vi "Return Hex Conversion 05.VI"(9 "Input Array":string[](array[string])) -> (0 "Value str":string, 1 "Calculated Chksum":u8 format="%02x", 2 "Vakue num":dbl format="%.2f", 3 "Description":string, 4 "Checksum Error":bool)   [LabVIEW 2023]
doc: "Converts Neslab return Hex String into comprehensible numbers and functions for display on the main interface."
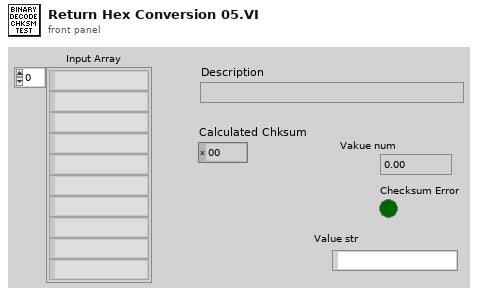
[diagram p1: front panel]
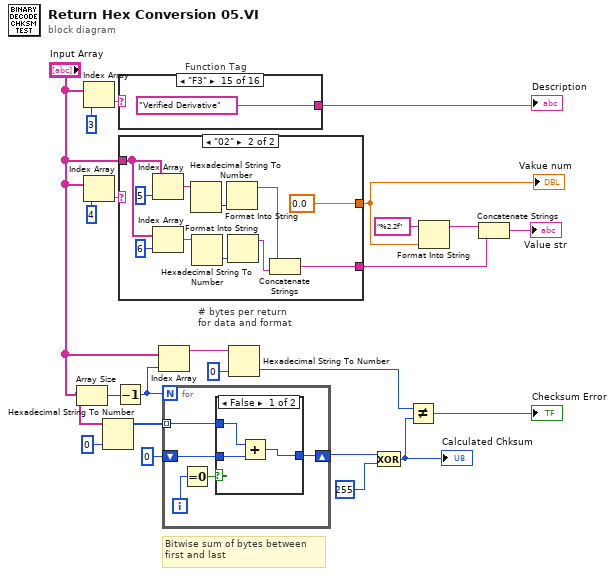
[diagram p0: block diagram]
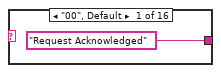
[diagram p3: hidden frame]
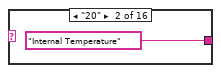
[diagram p4: hidden frame]
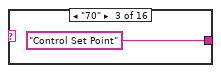
[diagram p5: hidden frame]
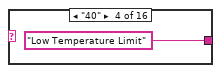
[diagram p6: hidden frame]
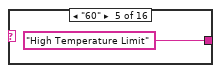
[diagram p7: hidden frame]
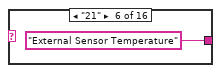
[diagram p8: hidden frame]
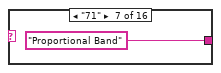
[diagram p9: hidden frame]
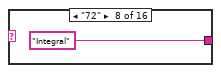
[diagram p10: hidden frame]
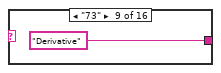
[diagram p11: hidden frame]
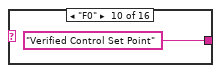
[diagram p12: hidden frame]
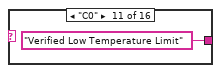
[diagram p13: hidden frame]
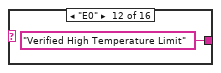
[diagram p14: hidden frame]
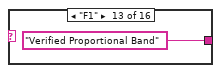
[diagram p15: hidden frame]
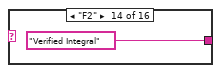
[diagram p16: hidden frame]
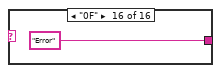
[diagram p17: hidden frame]
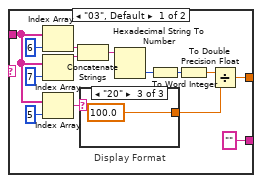
[diagram p18: hidden frame]
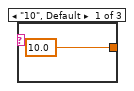
[diagram p19: hidden frame]
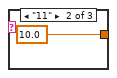
[diagram p20: hidden frame]
diagram:
  # "Bitwise sum of bytes between \nfirst and last"
  # "# bytes per return\nfor data and format"
  # "Function Tag"
  n1 = Array Size(array="Input Array") -> (size(s)=w13:i32)
  n2 = Index Array(array="Input Array", index=3 ("Index")) -> (element=w21:string)
  n3 = Index Array(array="Input Array", index=4 ("Index")) -> (element=w20:string)
  n4 = Hexadecimal String To Number(string="Input Array", default (0uL)=u8 0 ("default (0 U32)")) -> (number=w12:u8[])  [unwired: 1 in, 1 out]
  n5 = Decrement(x=w13) -> (x-1=w7:i32)
  n6 = case shown="\"F3\"" w21 {
    tunnel: ["Request Acknowledged" "Internal Temperature" "Control Set Point" "Low Temperature Limit" "High Temperature Limit" "External Sensor Temperature" "Proportional Band" "Integral" "Derivative" "Verified Control Set Point" "Verified Low Temperature Limit" "Verified High Temperature Limit" "Verified Proportional Band" "Verified Integral" "Verified Derivative" "Error"] -> w17
    frame "00", Default {
    }
    frame "20" {
    }
    frame "70" {
    }
    frame "40" {
    }
    frame "60" {
    }
    frame "21" {
    }
    frame "71" {
    }
    frame "72" {
    }
    frame "73" {
    }
    frame "F0" {
    }
    frame "C0" {
    }
    frame "E0" {
    }
    frame "F1" {
    }
    frame "F2" {
    }
    frame "F3" {
    }
    frame "0F" {
    }
  }
  "Description" <- w17
  n7 = case shown="\"02\"" w20 {
    tunnel: [w46 0.0] -> w15
    tunnel: ["" w65] -> w16
    tunnel: "Input Array" -> [w45 w57]
    frame "03", Default {
      # "Display Format"
      n8 = Index Array(array=w45, index=6 ("Index")) -> (element=w43:string)
      n9 = Index Array(array=w45, index=7 ("Index")) -> (element=w42:string)
      n10 = Index Array(array=w45, index=5 ("Index")) -> (element=w44:string)
      n11 = Concatenate Strings(w43, w42) -> (w50:string)
      n12 = case shown="\"20\"" w44 {
        tunnel: [10.0 10.0 100.0] -> w48
        frame "10", Default {
        }
        frame "11" {
        }
        frame "20" {
        }
      }
      n13 = Hexadecimal String To Number(string=w50) -> (number=w49:u32)  [unwired: 2 in, 1 out]
      n14 = To Word Integer(number=w49) -> (16bit integer=w41:i16)
      n15 = To Double Precision Float(number=w41) -> (double precision float=w47:dbl)
      n16 = Divide(x=w47, y=w48) -> (x/y=w46:dbl)
    }
    frame "02" {
      n17 = Index Array(array=w57, index=5 ("Index")) -> (element=w60:string)
      n18 = Index Array(array=w57, index=6 ("Index")) -> (element=w58:string)
      n19 = Hexadecimal String To Number(string=w60) -> (number=w59:u32)  [unwired: 2 in, 1 out]
      n20 = Hexadecimal String To Number(string=w58) -> (number=w62:u32)  [unwired: 2 in, 1 out]
      n21 = Format Into String(w59) -> (resulting string=w63:string)  [unwired: 3 in, 1 out]
      n22 = Format Into String(w62) -> (resulting string=w61:string)  [unwired: 3 in, 1 out]
      n23 = Concatenate Strings(w63, w61) -> (w65:string)
    }
  }
  "Vakue num" <- w15
  n24 = Index Array(array="Input Array", index=w7) -> (element=w4:string)
  n25 = for {
    N: w7 -> [_]
    tunnel: w12 -> [w70] mode=indexing
    shift-right: [w68] -> w8
    shift-left: u8 0 -> [w69]
    i -> [w72]
    n26 = Equal To 0?(x=w72) -> (x = 0?=w71:bool)
    n27 = case shown="False" w71 {
      tunnel: w70 -> [w74 _]
      tunnel: w69 -> [w75 w76]
      tunnel: [w73 w76] -> w68
      frame False {
        n28 = Add(x=w74, y=w75) -> (x+y=w73:u8)
      }
      frame True {
      }
    }
  }
  n29 = Hexadecimal String To Number(string=w4, default (0uL)=u8 0 ("default (0 U32)")) -> (number=w2:u8)  [unwired: 1 in, 1 out]
  n30 = Exclusive Or(1:u8 255 ("y"), 2:w8) -> (0:w3:u8)
  "Calculated Chksum" <- w3
  n31 = Not Equal?(x=w2, y=w3) -> (x != y?=→"Checksum Error":bool)
  n32 = Format Into String(format string="%2.2f" ("Format String"), w15) -> (resulting string=w18:string)  [unwired: 2 in, 1 out]
  n33 = Concatenate Strings(w18, w16) -> (→"Value str":string)
